vi "hydraharp_close_stream.vi"(8 "error in (no error)":errorcluster, 11 "hydraharp in":refnum<class "hydraharp.lvclass">) -> (0 "error out":errorcluster, 3 "hydraharp out":refnum<class "hydraharp.lvclass">)   [LabVIEW 2015, in "hydraharp.lvclass"]
uses:
  hydraharp.lvclass
  hydraharp.lvclass/hydraharp.ctl
  Data Logger Class/data_logger.lvclass
  hhlib.dll
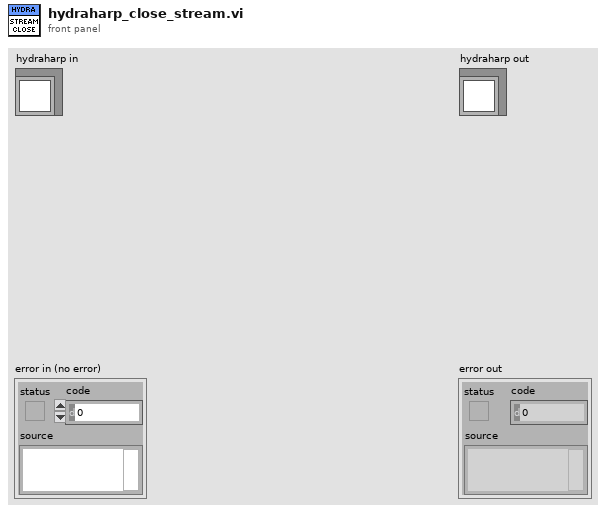
[diagram p1: front panel]
types:
  T1 = cluster{"log_bin_edges":dbl[], "ch1_photons":dbl[], "ch2_photons":dbl[], "elements_in_record_buffers":i32[], "number_of_new_photons":i32[]}
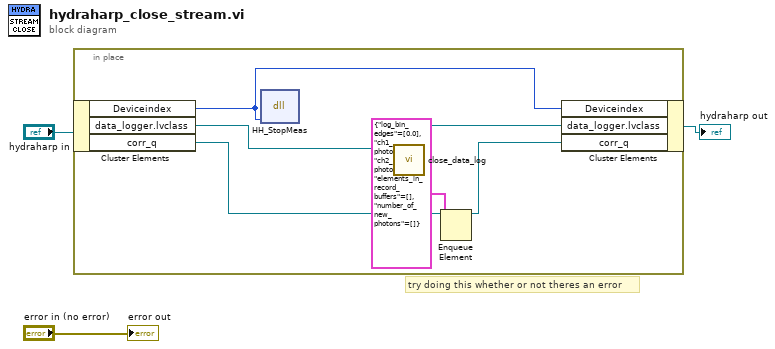
[diagram p0: block diagram]
diagram:
  # "try doing this whether or not theres an error"
  n1 = in-place {
    n2 = in-place-cluster #1("hydraharp in") -> ("Deviceindex"=w9:i32, "data_logger.lvclass"=w8:refnum<class "data_logger.lvclass">, "corr_q"=w6:refnum<queue>)
    n3 = dll-call lib="hhlib.dll" fn="HH_StopMeas"("devidx"=w9) -> ()  [unwired: 5 in, 2 out]
    n4 = call-dynamic "close_data_log.vi"("data_logger in"=w8) -> ("data_logger out"=w7:refnum<class "data_logger.lvclass">)  [unwired: 9 in, 1 out]
    n5 = Enqueue Element(queue=w6, element=T1 {"log_bin_edges"=[0.0], "ch1_photons"=[], "ch2_photons"=[], "elements_in_record_buffers"=[], "number_of_new_photons"=[]}) -> (queue out=w4:refnum<queue>)  [unwired: 2 in, 2 out]
    n6 = in-place-cluster #1("Deviceindex"=w9, "data_logger.lvclass"=w7, "corr_q"=w4) -> (→"hydraharp out":refnum<class "hydraharp.lvclass">)
  }
  "error out" <- "error in (no error)"
